vi "AddParamChannels.vi"(4 "Called From SysDef API (F)":bool, 5 "Parm Page GUID":string="11250030-7C42-42CF-BB8B-798981AF63E1", 6 "Type":T3, 7 "Default Message Data":u16[](array[numeric]), 8 "error in":errorcluster, 9 "Initial Value":dbl, 10 "Parameters to add":T2[](array[typedef]), 11 "Node Ref In":T1=18446744073709551615 format="%.0x") -> (0 "error out":errorcluster, 3 "Node Ref Out":T1=18446744073709551615 format="%.0x")   [LabVIEW 2011, in "AIT 1553 Custom Device.lvlib"]
uses:
  AIT 1553 Custom Device.lvlib
  <vilib>/NI Veristand/Custom Device API/Custom Device Item Ref.ctl
  <vilib>/NI Veristand/Custom Device API/Custom Device Channel Type.ctl
  Controls/1553 Param.ctl
  <vilib>/NI Veristand/Custom Device API/Custom Device Channel.ctl
  Controls and Global/Global.vi
  <vilib>/NI Veristand/Custom Device API/Custom Device API.lvlib
panel:
  # "xxxx delete this and fix up!"
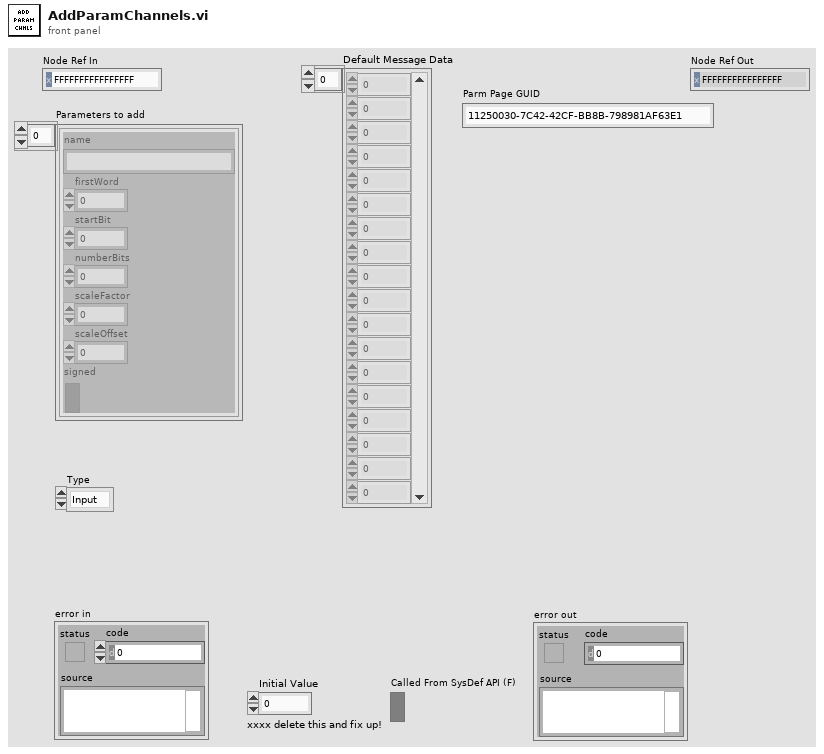
[diagram p1: front panel]
types:
  T1 = typedef "Custom Device API.lvlib/Custom Device Item Ref.ctl" = u64
  T2 = typedef "AIT 1553 Custom Device.lvlib/1553 Param.ctl" = cluster{"name":string, "firstWord":i32, "startBit":i32, "numberBits":i32, "scaleFactor":dbl, "scaleOffset":dbl, "signed":bool}
  T3 = typedef "Custom Device API.lvlib/Custom Device Channel Type.ctl" = enum16{"Input", "Output"}
  T4 = typedef "Custom Device API.lvlib/Custom Device Channel.ctl" = cluster{"Type":T3, "Units":string, "Default Value":dbl, "Faultable":bool, "Scalable":bool}
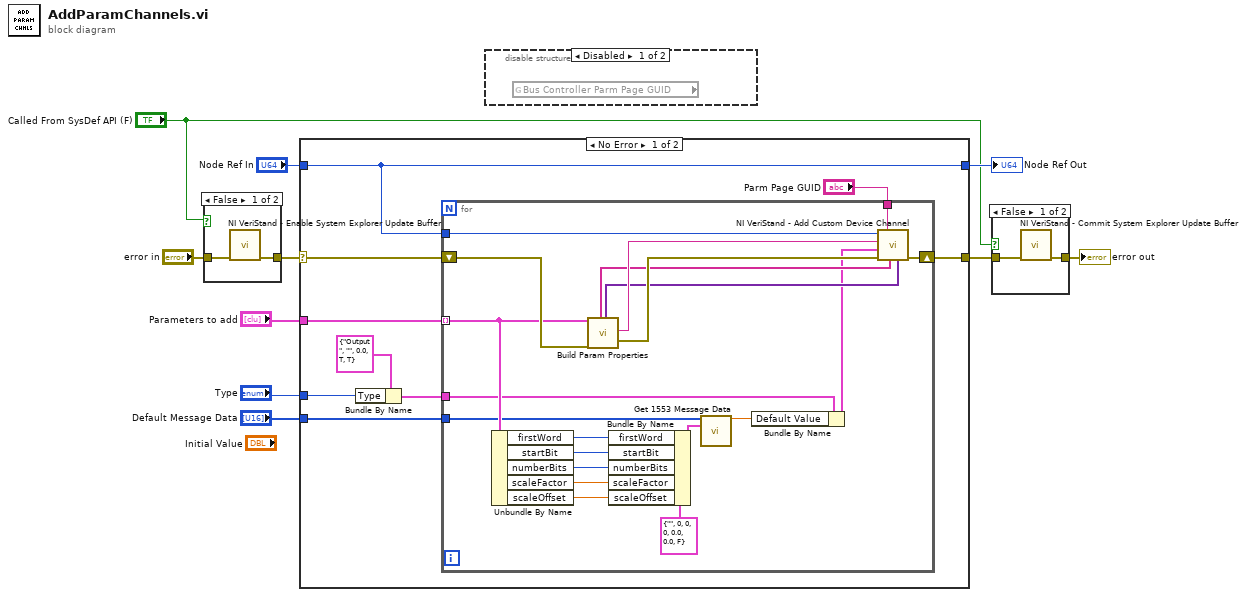
[diagram p0: block diagram]
diagram:
  n1 = case shown="False" "Called From SysDef API (F)" {
    tunnel: "error in" -> [w12 w13]
    tunnel: [w11 w13] -> w2
    frame False {
      n2 = call <vilib>:"NI VeriStand - Enable System Explorer Update Buffer.vi"("error in (no error)"=w12) -> ("error out"=w11:errorcluster)  [unwired: 10 in]
    }
    frame True {
    }
  }
  n3 = case shown="No Error" w2 {
    selector: w2 -> [w17 w44]
    tunnel: "Parameters to add" -> [w20 _]
    tunnel: "Node Ref In" -> [w16 w43]
    tunnel: "Type" -> [w19 _]
    tunnel: [w18 w44] -> w5
    tunnel: [w16 w43] -> w7
    tunnel: "Default Message Data" -> [w15 _]
    frame No Error {
      n4 = Bundle By Name(cluster=T4 {"Type"=enum."Output", "Units"="", "Default Value"=0.0, "Faultable"=TRUE, "Scalable"=TRUE} ("Channel"), "Type"=w19) -> (w22:T4)
      n5 = for {
        shift-right: [w42] -> w18
        shift-left: w17 -> [w39]
        tunnel: w16 -> [w41]
        tunnel: w22 -> [w24]
        tunnel: "Parm Page GUID" -> [w40]
        tunnel: w20 -> [w34] mode=indexing
        tunnel: w15 -> [w25]
        n6 = Unbundle By Name(w34) -> ("firstWord"=w27:i32, "startBit"=w28:i32, "numberBits"=w29:i32, "scaleFactor"=w30:dbl, "scaleOffset"=w31:dbl)
        n7 = call "Build Param Properties.vi"("1553 Parameter"=w34, "error in (no error)"=w39) -> ("Prop Names"=w36:string[], "Prop Values"=w35:variant[], "name"=w37:string, "error out"=w38:errorcluster)  [unwired: 9 in, 5 out]
        n8 = Bundle By Name(cluster=T2 {"name"="", "firstWord"=0, "startBit"=0, "numberBits"=0, "scaleFactor"=0.0, "scaleOffset"=0.0, "signed"=FALSE} ("1553 Parameter"), "firstWord"=w27, "startBit"=w28, "numberBits"=w29, "scaleFactor"=w30, "scaleOffset"=w31) -> (w26:T2)
        n9 = call "Get 1553 Message Data.vi"("MSG DATA"=w25, "1553 Parameter"=w26) -> ("Value"=w33:dbl)  [unwired: 12 in, 1 out]
        n10 = Bundle By Name(cluster=w24, "Default Value"=w33) -> (w23:T4)
        n11 = call <vilib>:"NI VeriStand - Add Custom Device Channel.vi"("Property Values"=w35, "Property names"=w36, "GUID (Default Channel)"=w40, "error in (no error)"=w38, "Channel"=w23, "Channel Name"=w37, "Parent Ref in"=w41) -> ("error out"=w42:errorcluster)  [unwired: 1 in, 3 out]
      }
    }
    frame Error {
    }
  }
  "Node Ref Out" <- w7
  n12 = disable-structure shown="Disabled" {
    frame Disabled {
      n13 = global read "Global.vi" "Bus Controller Parm Page GUID"() -> ()  [unwired: 1 out]
    }
    frame Enabled {
    }
  }
  n14 = case shown="False" "Called From SysDef API (F)" {
    tunnel: w5 -> [w46 w47]
    tunnel: [w45 w47] -> w4
    frame False {
      n15 = call <vilib>:"NI VeriStand - Commit System Explorer Update Buffer.vi"("error in (no error)"=w46) -> ("error out"=w45:errorcluster)  [unwired: 10 in]
    }
    frame True {
    }
  }
  "error out" <- w4
